vi "FPGA Main.vi"() -> ()   [LabVIEW 2013]
doc: "\"FPGA Main VI\"包含并列的一个控制循环和一个RT watchdog循环。\n－ 控制循环对4路输入通道并行地进行控制计算，将结果输出至输出通道。\n－RT Watchdog检查来自\"RT Main VI\"的周期触发，以确保RT与FPGA的通信正常。"
uses:
  <vilib>/rvi/Emulation/niFpgaSctlEmulationGetInTimedLoop.vi
  <vilib>/rvi/Emulation/niFpgaEmulationReportErrorSimple.vi
  <vilib>/rvi/Emulation/niFpgaGetClockAttributes.vi
  <vilib>/rvi/eio/common/nirviEmuTemplateMethod_errors.vi
  <vilib>/rvi/Emulation/niFpgaProcessEmulError.vi
  <vilib>/rvi/interface/RandomDataEmulation/nirviRandomDataFPGAFIFO.vi
  <vilib>/rvi/interface/RandomDataEmulation/niFpgaRandomDataHandleErrors.vi
  <vilib>/rvi/Emulation/niFpgaCriticalErrorInLSC.vi
  <vilib>/eio/EIONode/EIONode.xnode
  <vilib>/rvi/DataTransferAndStorage/Container/XNode/niFpgaContainer.xnode
  <vilib>/rvi/interface/RandomDataEmulation/nirviRandomDataFpgaReadWriteTemplate.vi
panel:
  out "FPGA Error":errorcluster caption="FPGA错误"
  out "Finished":bool caption="完成"
  in  "Stop":bool caption="停止"
  out "Module Underflow":bool caption="模块下溢"
  out "DMA FIFO Full":bool caption="DMA FIFO已满"
  out "Different Channel Count":bool caption="不同通道计数"
  out "Actual Loop Period (ticks)":u32 caption="实际循环周期"
  out "First Read":bool caption="首次读"
  in  "Number of Channels":i32=4 caption="通道数"
  in  "Channel Scale Array":fxp<+,24,12>[](array[numeric])=[1.0, 1.0, 1.0, 1.0] caption="换算数组"
  # "输入设置"
  # "状态监控"
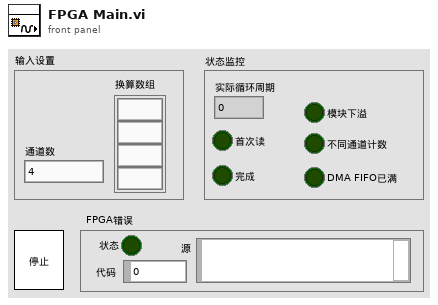
[diagram p1: front panel]
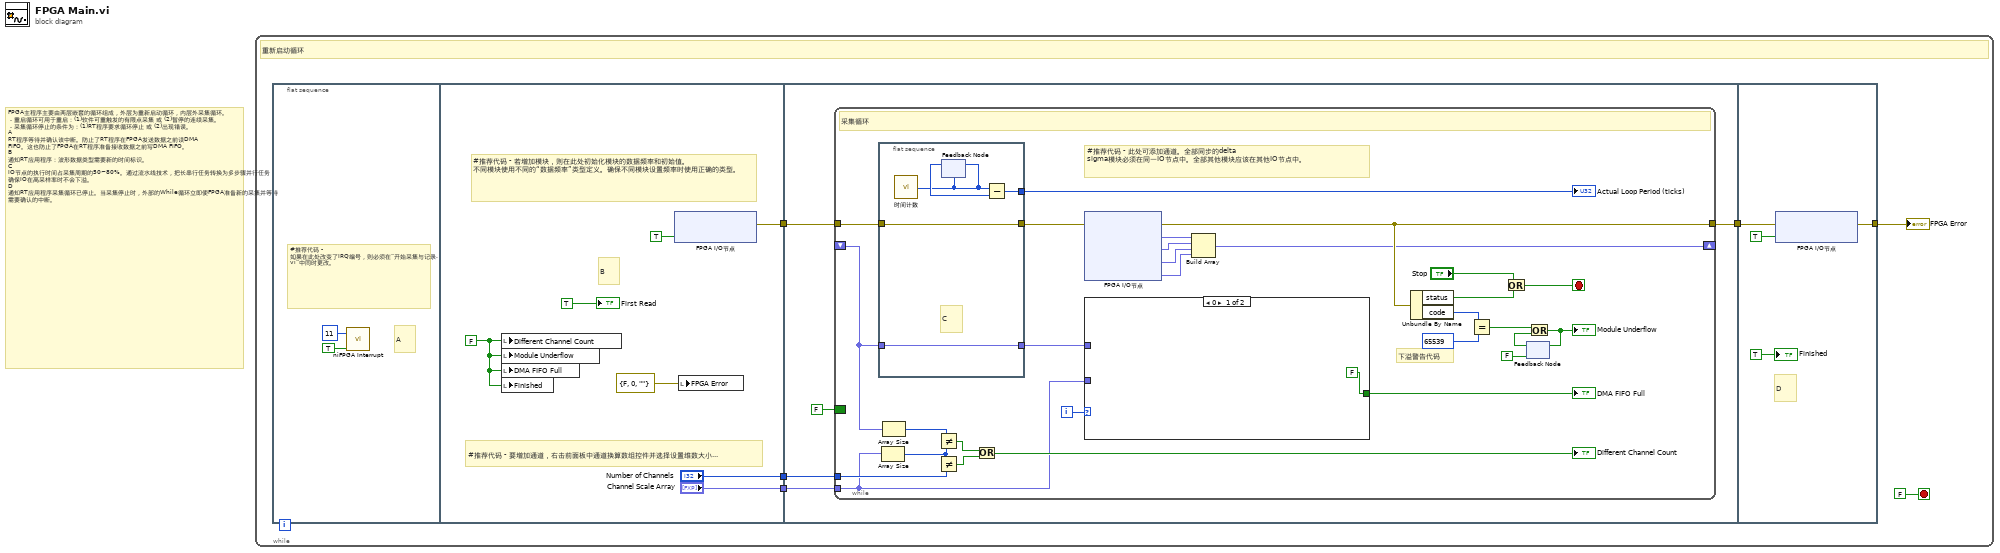
[diagram p0: block diagram]
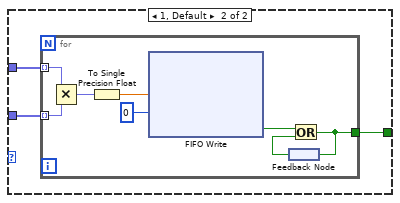
[diagram p2: hidden frame]
diagram:
  # "FPGA主程序主要由两层嵌套的循环组成，外层为重新启动循环，内层外采集循环。\n－重启循环可用于重启：(1)软件可重触发的有限点采集 或 (2)暂停的连续采集。\n－采集循环停止的条件为：(1)RT程序要求循环停止 或 (2)出现错误。 \nA\nRT程序等待并确认该中断。防止了RT程序在FPGA发送数据之前读DMA FIFO。这也防止了FPGA在RT程序准备接收数据之前写DMA FIFO。\nB\n通知RT应用程序：波形数据类型需要新的时间标识。\nC\nIO节点的执行时间占采集周期的50~80%。通过流水线技术，把长串行任务转换为多步骤并行任务，确保IO在高采样率时不会下溢。\nD\n通知RT应用程序采集循环已停止。当采集停止时，外部的While循环立即使FPGA准备新的采集并等待需要确认的中断。"
  n1 = while {
    stop <- FALSE stop-if-true
    # "重新启动循环"
    n2 = flat-sequence {
      tunnel: [w15] -> w6
      tunnel: ["Channel Scale Array"] -> w5
      tunnel: ["Number of Channels"] -> w1
      tunnel: w6 -> [w20]
      tunnel: w5 -> [w19]
      tunnel: [w18] -> w4
      tunnel: w1 -> [w16]
      tunnel: w4 -> [w68]
      tunnel: [w67] -> w3
      frame #0 {
        # "#推荐代码 - 如果在此处改变了IRQ编号，则必须在“开始采集与记录.vi”中同时更改。"
        # "A"
        n3 = call <vilib>:"niFPGA Interrupt.vi"("Wait Until Cleared (F)"=TRUE ("Wait Until Cleared"), "IRQ Number (0)"=u8 11 ("IRQ Number")) -> ()  [unwired: 1 in]
      }
      frame #1 {
        w12 = FALSE ("Module Underflow")
        # "B"
        # "#推荐代码 - 要增加通道，右击前面板中通道换算数组控件并选择设置维数大小..."
        # "#推荐代码 - 若增加模块，则在此处初始化模块的数据频率和初始值。\n不同模块使用不同的“数据频率”类型定义。确保不同模块设置频率时使用正确的类型。"
        n4 = local write "Different Channel Count"(w12) -> ()
        n5 = local write "Module Underflow"(w12) -> ()
        n6 = local write "DMA FIFO Full"(w12) -> ()
        n7 = local write "Finished"(w12) -> ()
        n8 = xnode "FPGA I/O节点"("Mod1/Start"=TRUE) -> ("错误输出"=w15:errorcluster)  [unwired: 2 in, 1 out]
        n9 = local write "FPGA Error"(errorcluster {"status"=FALSE, "code"=0, "source"=""} ("FPGA Error")) -> ()
        "First Read" <- TRUE ("First Read")
      }
      frame #2 {
        n10 = while {
          tunnel: w20 -> [w48]
          tunnel: [w33] -> w18
          shift-right: [w32] -> _
          shift-left: _ -> [w28]
          tunnel: w19 -> [w21]
          border: FALSE -> [_]
          tunnel: w16 -> [w24]
          i -> [w31]
          stop <- w49 stop-if-true
          # "下溢警告代码"
          # "#推荐代码 - 此处可添加通道。全部同步的delta sigma模块必须在同一IO节点中。全部其他模块应该在其他IO节点中。"
          # "采集循环"
          n11 = flat-sequence {
            tunnel: [w54] -> w47
            tunnel: w48 -> [w54]
            tunnel: [w50] -> w46
            tunnel: w28 -> [w53]
            tunnel: [w53] -> w30
            frame #0 {
              # "C"
              n12 = call "时间计数"() -> ("Tick Count(Ticks)"=w51:u32)
              n13 = feedback #1(w51) -> (w52:u32)
              n14 = feedback-in #1(w51) -> ()
              n15 = Subtract(x=w51, y=w52) -> (x-y=w50:u32)
            }
          }
          n16 = Array Size(array=w21) -> (size(s)=w25:i32)
          n17 = Array Size(array=w28) -> (size(s)=w39:i32)
          n18 = Not Equal?(x=w39, y=w25) -> (x != y?=w27:bool)
          n19 = Not Equal?(x=w25, y=w24) -> (x != y?=w22:bool)
          n20 = Or(x=w27, y=w22) -> (x .or. y?=→"Different Channel Count":bool)
          n21 = xnode "FPGA I/O节点"("错误输入"=w47) -> ("错误输出"=w33:errorcluster, "Mod1/AI0"=w45:fxp<+/-,24,4>, "Mod1/AI1"=w42:fxp<+/-,24,4>, "Mod1/AI2"=w44:fxp<+/-,24,4>, "Mod1/AI3"=w43:fxp<+/-,24,4>)  [unwired: 4 in, 4 out]
          n22 = case shown="0" w31 {
            tunnel: w30 -> [_ w58]
            tunnel: w21 -> [_ w57]
            tunnel: [FALSE w56] -> w29
            frame 0 {
            }
            frame 1, Default {
              n23 = for {
                tunnel: [w61] -> w56
                tunnel: w58 -> [w66] mode=indexing
                tunnel: w57 -> [w65] mode=indexing
                n24 = Multiply(x=w66, y=w65) -> (x*y=w64:fxp<+/-,48,16>)
                n25 = To Single Precision Float(number=w64) -> (single precision float=w63:sgl)
                n26 = xnode ("FIFO Write")("元素"=w63, "超时"=0) -> ("超时？"=w62:bool)  [unwired: 1 in, 1 out]
                n27 = feedback #2() -> (w60:bool)
                n28 = Or(x=w62, y=w60) -> (x .or. y?=w61:bool)
                n29 = feedback-in #2(w61) -> ()
              }
            }
          }
          "DMA FIFO Full" <- w29
          n30 = Build Array(w45, w42, w44, w43) -> (w32:fxp<+/-,24,4>[])
          n31 = Unbundle By Name(w33) -> ("status"=w40:bool, "code"=w26:i32)
          n32 = Equal?(x=w26, y=65539) -> (x = y?=w38:bool)
          n33 = Or(x="Stop", y=w40) -> (x .or. y?=w49:bool)
          n34 = feedback #3 ("Latch")(FALSE) -> (w36:bool)
          n35 = Or(x=w38, y=w36) -> (x .or. y?=w34:bool)
          "Module Underflow" <- w34
          n36 = feedback-in #3(w34) -> ()
          "Actual Loop Period (ticks)" <- w46
        }
      }
      frame #3 {
        # "D"
        n37 = xnode "FPGA I/O节点"("错误输入"=w68, "Mod1/Stop"=TRUE) -> ("错误输出"=w67:errorcluster)  [unwired: 1 in, 1 out]
        "Finished" <- TRUE ("Finished")
      }
    }
    "FPGA Error" <- w3
  }
